vi "Actor Core.vi"(8 "error in":errorcluster, 11 "[V] Main UI in":refnum<class "[V] Main UI.lvclass">) -> (0 "error out":errorcluster, 3 "Actor out":refnum<class "Actor.lvclass">)   [LabVIEW 2020, in "[V] Main UI.lvlib" / "[V] Main UI.lvclass"]
doc: "(<B>Filename</B>: Actor Framework.lvlib:Actor.lvclass:Actor Core.vi)\n\nReceives messages to the actor, reacts to them, and initiates any error handling that may shut the actor down.\n\nDescendant classes may override this VI to append parallel tasks for the actor to complete while it handles messages. Overrides use the Call Parent Class Method node."
uses:
  [V] Main UI.lvclass
  C:/Program Files (x86)/National Instruments/LabVIEW 2020/vi.lib/ActorFramework/Actor/Actor.lvclass
  <vilib>/ActorFramework/Actor/Actor.lvclass
  Controls/Flat Config.ctl
  Controls/Backword.ctl
  Controls/Forward.ctl
  Controls/number.ctl
  <vilib>/Utility/miscctls.llb/LVBoundsTypeDef.ctl
  [V] Main UI.lvclass/[V] Main UI.ctl
  Depden On/Abstruct View/Abstruct View/Abstruct View.lvclass/Abstruct View.ctl
  <vilib>/ActorFramework/Actor/Actor.lvclass/Actor.ctl
  <vilib>/ActorFramework/Message Enqueuer/Message Enqueuer.lvclass/Message Enqueuer.ctl
  [V] Main UI Messages/Select Path Msg/Select Path Msg.lvclass/Select Path Msg.ctl
  <vilib>/ActorFramework/Message Enqueuer/Message Priority.ctl
  [V] Main UI Messages/Play Pause Msg/Play Pause Msg.lvclass/Play Pause Msg.ctl
  [V] Main UI Messages/Data View Display Msg/Data View Display Msg.lvclass/Data View Display Msg.ctl
  [V] Main UI Messages/Range Msg/Range Msg.lvclass/Range Msg.ctl
  Depden On/Abstruct View/Abstruct View/Data Accessors/Read Stop Event.vi
  Depden On/Abstruct View/Abstruct View/Data Accessors/Write Core VI.vi
  <vilib>/ActorFramework/Message Enqueuer/Init from Existing Queue.vi
  <vilib>/ActorFramework/Message Enqueuer/Enqueue.vi
  <vilib>/ActorFramework/Stop Msg/Stop Msg.lvclass
  C:/Program Files (x86)/National Instruments/LabVIEW 2020/vi.lib/ActorFramework/Message/Message.lvclass
  [V] Main UI Messages/Select Path Msg/Select Path Msg.lvclass
  [V] Main UI Messages/Play Pause Msg/Play Pause Msg.lvclass
  [V] Main UI Messages/Next Frame Msg/Next Frame Msg.lvclass
  [V] Main UI Messages/Last Frame Msg/Last Frame Msg.lvclass
  [V] Main UI Messages/Launch Setting Msg/Launch Setting Msg.lvclass
  [V] Main UI Messages/Data View Display Msg/Data View Display Msg.lvclass
  [V] Main UI Messages/Range Msg/Range Msg.lvclass
  <vilib>/ActorFramework/Message Priority Queue/Priority Enqueue.vi
  <vilib>/ActorFramework/Message Enqueuer/Message Enqueuer.lvclass
  Depden On/MVVM Framework/MVVM Abstruct View/MVVM Abstruct View/MVVM Abstruct View.lvclass
panel:
  in  "Setting Boolean":T1
  in  "Table Button":bool
  in  "XY Chart":bool
  in  "Waveform Chart":bool
  in  "Range Silder":T2 scale=0.0..100.0
  in  "Forward":T3
  in  "Backward":T4
  in  "Run Pause":bool
  out "File Path":string
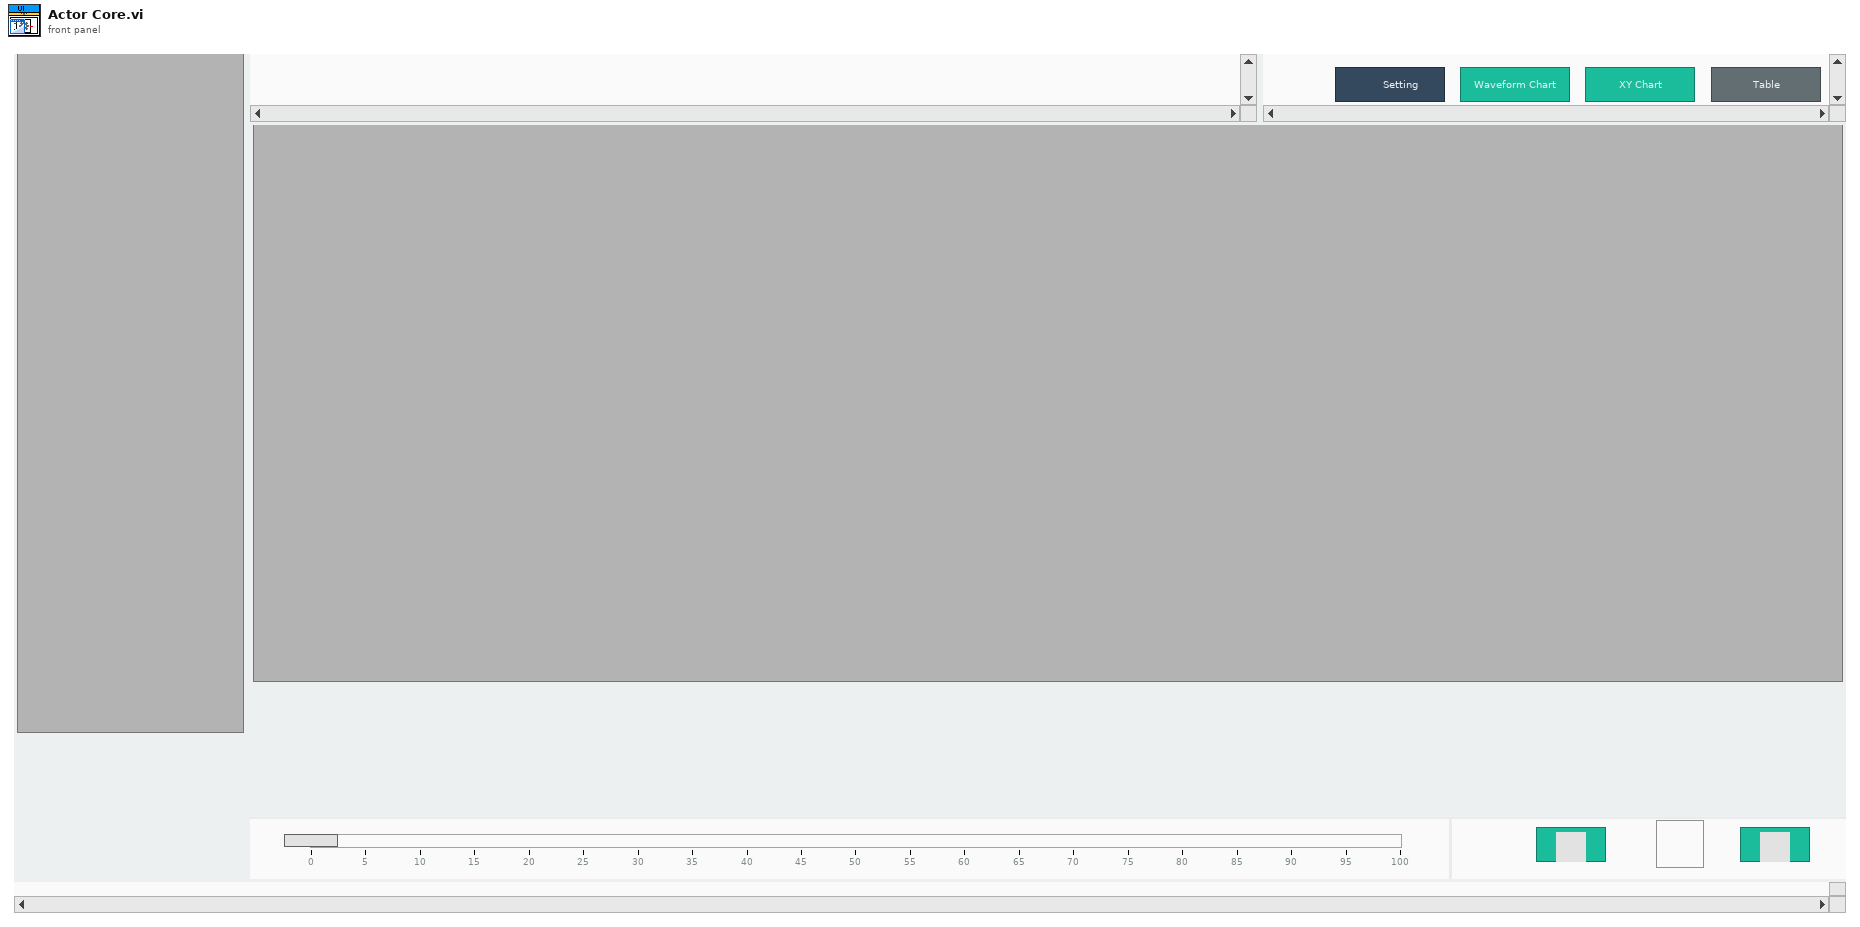
[diagram p1: front panel]
types:
  T1 = typedef "Flat Config.ctl" = bool
  T2 = typedef "number.ctl" = i8
  T3 = typedef "Forward.ctl" = bool
  T4 = typedef "Backword.ctl" = bool
  T5 = typedef "LVBoundsTypeDef.ctl" = cluster{"Width":u32, "Height":u32}
  T6 = typedef "Actor Framework.lvlib/Message Enqueuer.lvclass/Message Priority.ctl" = enum16{"Low", "Normal", "High"}
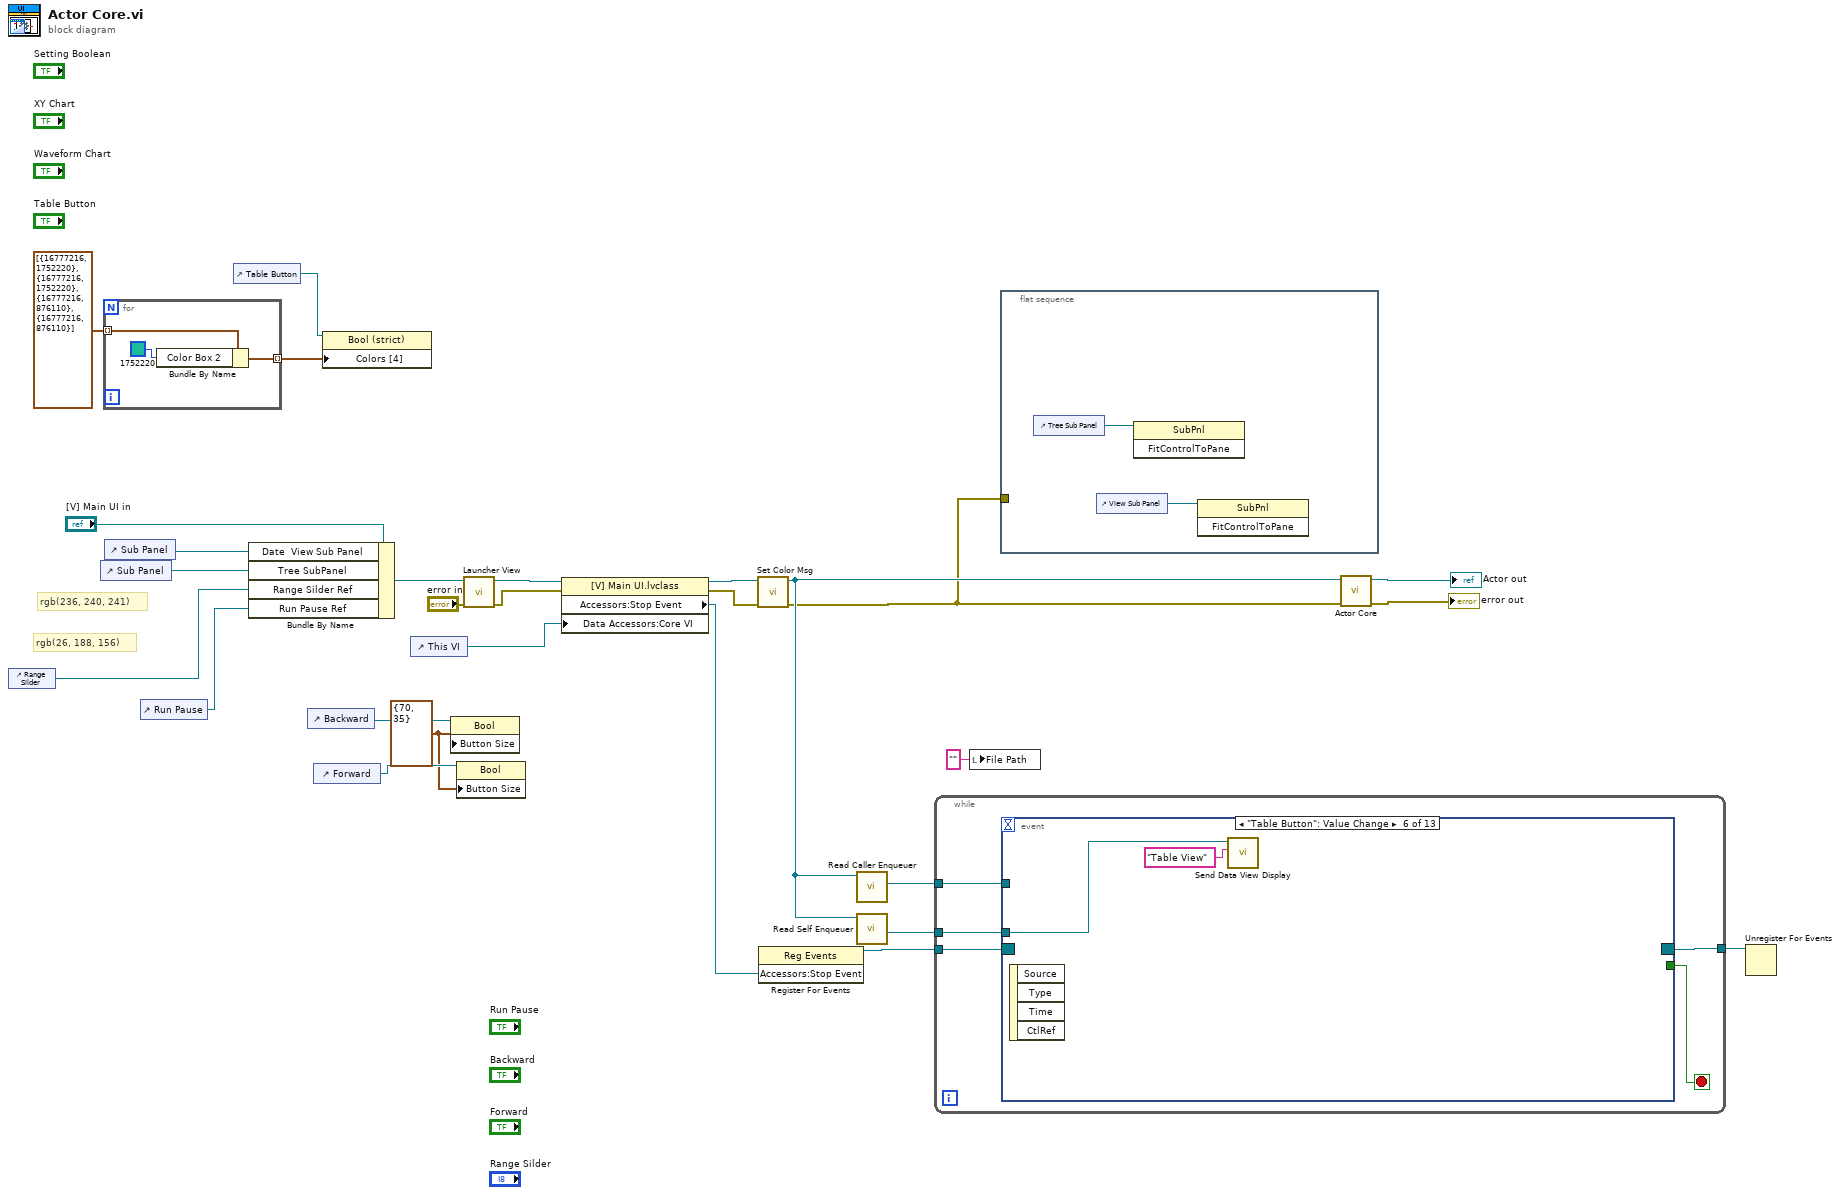
[diagram p0: block diagram]
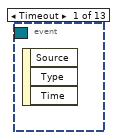
[diagram p2: hidden frame]
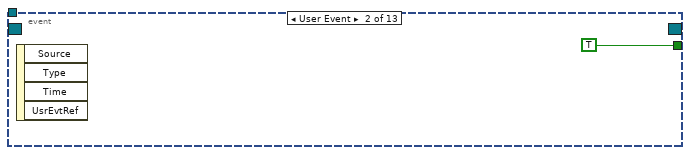
[diagram p3: hidden frame]
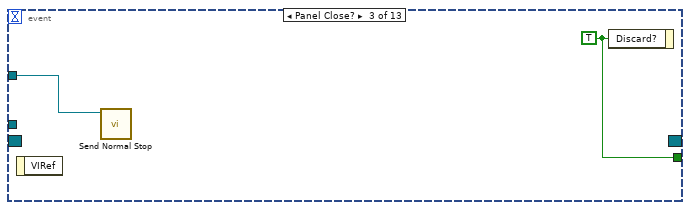
[diagram p4: hidden frame]
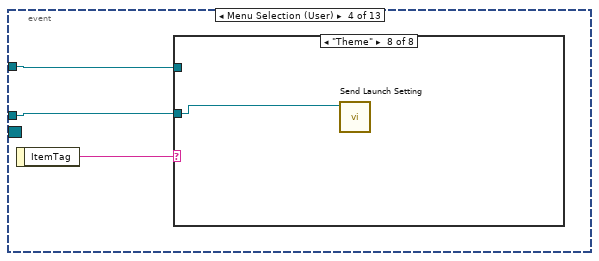
[diagram p5: hidden frame]
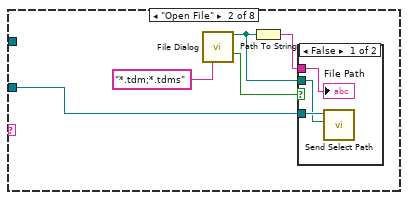
[diagram p7: hidden frame]
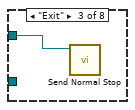
[diagram p9: hidden frame]
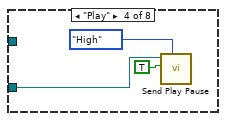
[diagram p10: hidden frame]
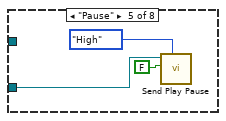
[diagram p11: hidden frame]
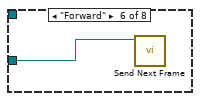
[diagram p12: hidden frame]
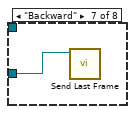
[diagram p13: hidden frame]
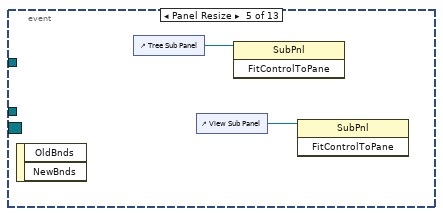
[diagram p14: hidden frame]
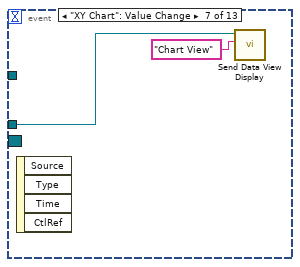
[diagram p15: hidden frame]
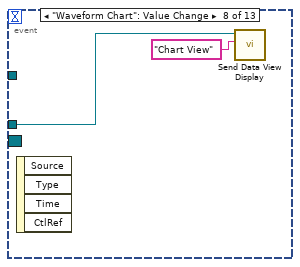
[diagram p16: hidden frame]
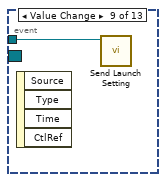
[diagram p17: hidden frame]
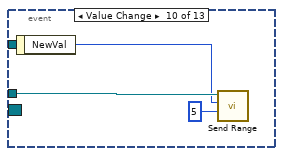
[diagram p18: hidden frame]
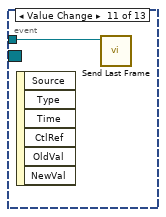
[diagram p19: hidden frame]
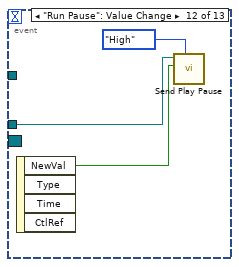
[diagram p20: hidden frame]
diagram:
  w1 = T5 {"Width"=70, "Height"=35} ("Button Size")
  # "rgb(26, 188, 156)"
  # "rgb(236, 240, 241)"
  n1 = control-ref of="Range Silder"() -> (w5:refnum<vi>)
  n2 = control-ref of="Sub Panel"() -> (w11:refnum<vi>)
  n3 = for {
    tunnel: cluster{"Color Box":u32, "Color Box 2":u32}[] [{"Color Box"=16777216, "Color Box 2"=1752220}, {"Color Box"=16777216, "Color Box 2"=1752220}, {"Color Box"=16777216, "Color Box 2"=876110}, {"Color Box"=16777216, "Color Box 2"=876110}] ("Colors [4]") -> [w31] mode=indexing
    tunnel: [w29] -> w21 mode=indexing
    n4 = Bundle By Name(cluster=w31, "Color Box 2"=u32 1752220) -> (w29:cluster{"Color Box":u32, "Color Box 2":u32})
  }
  n5 = control-ref of="Sub Panel"() -> (w10:refnum<vi>)
  n6 = control-ref of="Run Pause"() -> (w9:refnum<vi>)
  n7 = control-ref of="Table Button"() -> (w23:refnum<vi>)
  n8 = Bundle By Name(cluster="[V] Main UI in", "Date  View Sub Panel"=w10, "Tree SubPanel"=w11, "Range Silder Ref"=w5, "Run Pause Ref"=w9) -> (w19:refnum<class "[V] Main UI.lvclass">)
  n9 = control-ref of="Backward"() -> (w3:refnum<vi>)
  n10 = control-ref of="Forward"() -> (w2:refnum<vi>)
  n11 = property class="Bool (strict)"(reference=w23, "Colors [4]"=w21) -> ()  [unwired: 1 in, 2 out]
  n12 = control-ref of="This VI"() -> (w12:refnum<vi>)
  n13 = property class="Bool"(reference=w3, "Button Size"=w1) -> ()  [unwired: 1 in, 2 out]
  n14 = property class="Bool"(reference=w2, "Button Size"=w1) -> ()  [unwired: 1 in, 2 out]
  n15 = call "Launcher View.vi"("error in (no error)"="error in", "[V] Main UI in"=w19) -> ("error out"=w17:errorcluster, "[V] Main UI out"=w18:refnum<class "[V] Main UI.lvclass">)  [unwired: 8 in]
  n16 = property class="[V] Main UI.lvclass"(reference=w18, error in=w17, "Data Accessors:Core VI"=w12) -> (reference out=w15:refnum<class "[V] Main UI.lvclass">, error out=w14:errorcluster, "Accessors:Stop Event"=w26:refnum<user-event>)
  n17 = call "Set Color Msg.vi"("error in (no error)"=w14, "[V] Main UI in"=w15) -> ("error out"=w6:errorcluster, "[V] Main UI out"=w8:refnum<class "[V] Main UI.lvclass">)  [unwired: 8 in]
  n18 = register-events(w26) -> (reference out=w25:refnum<event-registration>)  [unwired: 2 in, 1 out]
  n19 = call <vilib>:"Read Caller Enqueuer.vi"("Actor"=w8) -> ("Caller Enqueuer"=w7:refnum<class "Message Enqueuer.lvclass">)  [unwired: 10 in]
  n20 = call <vilib>:"Read Self Enqueuer.vi"("Actor"=w8) -> ("Self Enqueuer"=w16:refnum<class "Message Enqueuer.lvclass">)  [unwired: 10 in]
  n21 = while {
    tunnel: w25 -> [w36]
    tunnel: [w35] -> w24
    tunnel: w16 -> [w33]
    tunnel: w7 -> [w32]
    stop <- w34 stop-if-true
    n22 = event shown="[5] \"Table Button\": Value Change" {
      selector: w36 -> [_ _ _ _ _ _ _ _ _ _ _ _ _]
      dyn-events: [_ _ _ _ _ _ _ _ _ _ _ _ _] -> w35
      timeout: _ -> [_ _ _ _ _ _ _ _ _ _ _ _ _]
      tunnel: [_ TRUE w39 _ _ _ _ _ _ _ _ _ _] -> w34
      tunnel: w33 -> [_ _ _ w42 _ w64 w66 w68 w69 w72 w73 w75 w77]
      tunnel: w32 -> [_ _ w38 w40 _ _ _ _ _ _ _ _ _]
      event Timeout {
        n23 = event-data() -> ()  [unwired: 1 in, 3 out]
      }
      event User Event {
        n24 = event-data() -> ()  [unwired: 1 in, 4 out]
      }
      event Panel Close? {
        w39 = TRUE ("Discard?")
        n25 = event-data() -> ()  [unwired: 1 in, 1 out]
        n26 = call <vilib>:"Send Normal Stop.vi"("Message Enqueuer"=w38) -> ()  [unwired: 10 in, 1 out]
        n27 = event-data("Discard?"=w39) -> ()  [unwired: 1 in, 1 out]
      }
      event Menu Selection (User) {
        n28 = event-data() -> ("ItemTag"=w41:string)  [unwired: 1 in]
        n29 = case shown="\"Theme\"" w41 {
          tunnel: w42 -> [_ w47 _ w53 w56 w58 w59 w60]
          tunnel: w40 -> [_ _ w51 _ _ _ _ _]
          frame "False", Default {
          }
          frame "Open File" {
            n30 = call "File Dialog"("pattern (all files)"="*.tdm;*.tdms") -> ("selected path"=w44:path, "cancelled"=w45:bool)  [unwired: 11 in, 2 out]
            n31 = Path To String(path=w44) -> (string=w43:string)
            n32 = case shown="False" w45 {
              tunnel: w47 -> [w50 _]
              tunnel: w44 -> [w49 _]
              tunnel: w43 -> [w48 _]
              frame False {
                n33 = call "Send Select Path.vi"("File Path"=w49, "Message Enqueuer"=w50) -> ()  [unwired: 8 in, 2 out]
                "File Path" <- w48
              }
              frame True {
              }
            }
          }
          frame "Exit" {
            n34 = call <vilib>:"Send Normal Stop.vi"("Message Enqueuer"=w51) -> ()  [unwired: 10 in, 1 out]
          }
          frame "Play" {
            n35 = call "Send Play Pause.vi"("Message Priority (Normal)"=Message_Priority."High", "Play Pause"=TRUE, "Message Enqueuer"=w53) -> ()  [unwired: 7 in, 2 out]
          }
          frame "Pause" {
            n36 = call "Send Play Pause.vi"("Message Priority (Normal)"=Message_Priority."High", "Play Pause"=FALSE, "Message Enqueuer"=w56) -> ()  [unwired: 7 in, 2 out]
          }
          frame "Forward" {
            n37 = call "Send Next Frame.vi"("Message Enqueuer"=w58) -> ()  [unwired: 9 in, 2 out]
          }
          frame "Backward" {
            n38 = call "Send Last Frame.vi"("Message Enqueuer"=w59) -> ()  [unwired: 9 in, 2 out]
          }
          frame "Theme" {
            n39 = call "Send Launch Setting.vi"("Message Enqueuer"=w60) -> ()  [unwired: 9 in, 2 out]
          }
        }
      }
      event Panel Resize {
        n40 = event-data() -> ()  [unwired: 1 in, 2 out]
        n41 = control-ref of="Tree Sub Panel"() -> (w61:refnum<vi>)
        n42 = control-ref of="View Sub Panel"() -> (w62:refnum<vi>)
        n43 = invoke class="SubPnl" method="FitControlToPane"(reference=w61) -> ()  [unwired: 2 in, 3 out]
        n44 = invoke class="SubPnl" method="FitControlToPane"(reference=w62) -> ()  [unwired: 2 in, 3 out]
      }
      event "Table Button": Value Change {
        n45 = event-data() -> ()  [unwired: 1 in, 4 out]
        n46 = call "Send Data View Display.vi"("Name"="Table View", "Message Enqueuer"=w64) -> ()  [unwired: 8 in, 2 out]
      }
      event "XY Chart": Value Change {
        n47 = event-data() -> ()  [unwired: 1 in, 4 out]
        n48 = call "Send Data View Display.vi"("Name"="Chart View", "Message Enqueuer"=w66) -> ()  [unwired: 8 in, 2 out]
      }
      event "Waveform Chart": Value Change {
        n49 = event-data() -> ()  [unwired: 1 in, 4 out]
        n50 = call "Send Data View Display.vi"("Name"="Chart View", "Message Enqueuer"=w68) -> ()  [unwired: 8 in, 2 out]
      }
      event Value Change {
        n51 = event-data() -> ()  [unwired: 1 in, 4 out]
        n52 = call "Send Launch Setting.vi"("Message Enqueuer"=w69) -> ()  [unwired: 9 in, 2 out]
      }
      event Value Change {
        n53 = event-data() -> ("NewVal"=w70:T2)  [unwired: 1 in]
        n54 = call "Send Range.vi"("length"=u8 5 ("y"), "index"=w70, "Message Enqueuer"=w72) -> ()  [unwired: 7 in, 2 out]
      }
      event Value Change {
        n55 = event-data() -> ()  [unwired: 1 in, 6 out]
        n56 = call "Send Last Frame.vi"("Message Enqueuer"=w73) -> ()  [unwired: 9 in, 2 out]
      }
      event "Run Pause": Value Change {
        n57 = event-data() -> ("NewVal"=w76:bool)  [unwired: 1 in, 3 out]
        n58 = call "Send Play Pause.vi"("Message Priority (Normal)"=Message_Priority."High", "Play Pause"=w76, "Message Enqueuer"=w75) -> ()  [unwired: 7 in, 2 out]
      }
      event Value Change {
        n59 = event-data() -> ()  [unwired: 1 in, 6 out]
        n60 = call "Send Next Frame.vi"("Message Enqueuer"=w77) -> ()  [unwired: 9 in, 2 out]
      }
    }
  }
  n61 = local write "File Path"("" ("File Path")) -> ()
  n62 = flat-sequence {
    tunnel: w6 -> [_]
    frame #0 {
      n63 = control-ref of="Tree Sub Panel"() -> (w79:refnum<vi>)
      n64 = control-ref of="View Sub Panel"() -> (w78:refnum<vi>)
      n65 = invoke class="SubPnl" method="FitControlToPane"(reference=w79) -> ()  [unwired: 2 in, 3 out]
      n66 = invoke class="SubPnl" method="FitControlToPane"(reference=w78) -> ()  [unwired: 2 in, 3 out]
    }
  }
  n67 = call-parent "Actor Core.vi"("error in"=w6, "Abstruct View in"=w8) -> ("error out"=→"error out":errorcluster, "Actor out"=→"Actor out":refnum<class "Actor.lvclass">)  [unwired: 8 in]
  n68 = Unregister For Events(event registration refnum=w24) -> ()  [unwired: 1 in, 1 out]
